vi "Standard_Error_Est.vi"(2 "N":dbl, 3 "4th order moment u^4":dbl, 4 "2nd order moment u^2":dbl) -> (0 "Standard error in variance":dbl, 1 "Standard error in Mean":dbl)   [LabVIEW 2010]
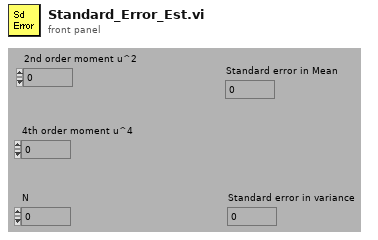
[diagram p1: front panel]
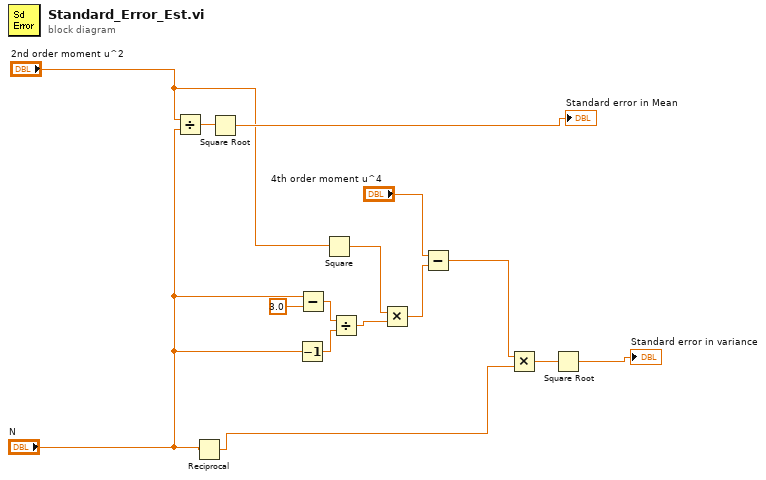
[diagram p0: block diagram]
diagram:
  n1 = Divide(x="2nd order moment u^2", y="N") -> (x/y=w15:dbl)
  n2 = Reciprocal(x="N") -> (1/x=w4:dbl)
  n3 = Square Root(x=w15) -> (sqrt(x)=→"Standard error in Mean":dbl)
  n4 = Decrement(x="N") -> (x-1=w11:dbl)
  n5 = Subtract(x="N", y=3.0) -> (x-y=w12:dbl)
  n6 = Square(x="2nd order moment u^2") -> (x^2=w8:dbl)
  n7 = Divide(x=w12, y=w11) -> (x/y=w10:dbl)
  n8 = Multiply(x=w8, y=w10) -> (x*y=w7:dbl)
  n9 = Subtract(x="4th order moment u^4", y=w7) -> (x-y=w5:dbl)
  n10 = Multiply(x=w5, y=w4) -> (x*y=w3:dbl)
  n11 = Square Root(x=w3) -> (sqrt(x)=→"Standard error in variance":dbl)
